vi "Demo - GNU Octave Terminal.vi"() -> ()   [LabVIEW 2020, in "GOLPI library.lvlib"]
doc: "Demontration of GOLPI: GNU Octave terminal.\n\n---\nGOLPI works only with lv_proc.dll library, which is part of vipm package or should be delivered together with packed library. Placement of this dll is selected in terminal of Start GNU Octave.vi."
uses:
  GOLPI library.lvlib
  GOLPI reference Type Def.ctl
  Pipe Handle.ctl
  LV Process library.lvlib
panel:
  in  "hide debug console":bool=TRUE
  out "debug data":T1(array[cluster])
  in  "debug mode\n(only nonempty buffers)":bool
  out "GOLPI ref. pipe":T2={"pipe handle"={"lv_proc.dll file path"=path "", "process instance handle"=[], "debug mode"=FALSE, "debug data"=[]}, "fast read timeout [ms]"=500, "fast read settle time [ms]"=10, "fast read to multiple [ms]"=1, "max elements per input line"=100, "slow read timeout [ms]"=500, "stdin double format specifier"="%_16e", "max elements per stdout output column"=100, "console mode bitstream"=FALSE, "bitstream first read timeout [ms]"=1000, "bitstream read timeout [ms]"=50, "struct transfer possible"=FALSE, "matlab mode"=FALSE}
  out "bytes remaining":i32
  in  "quit":bool
  out "GNU Octave running":bool
  out "read buffer":string
  in  "command buffer":string
  in  "command":bool
  out "objects after start":refnum<vi>[](array[refnum])
  out "objects before start":refnum<vi>[](array[refnum])
  in  "stop":bool
  out "error":errorcluster
  in  "start":bool
  in  "octave binary directory":path=path "C:/Program Files/Octave-3.6.2/bin"
  in  "working directory":path=path "C:/"
  out "exit code":i32
  out "GNU Octave version":string
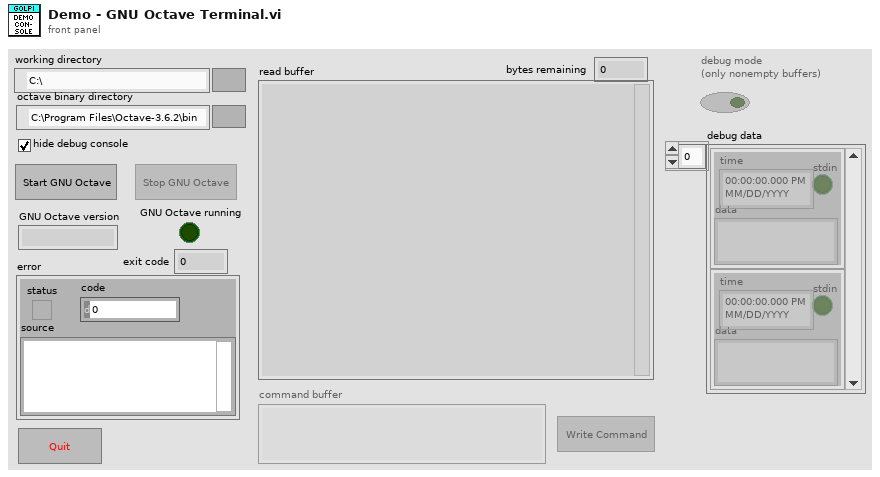
[diagram p1: front panel]
types:
  T1 = cluster{"time":timestamp, "stdin":bool, "data":string}[]
  T2 = typedef "GOLPI library.lvlib/GOLPI reference Type Def.ctl" = cluster{"pipe handle":T3, "fast read timeout [ms]":u32, "fast read settle time [ms]":u32, "fast read to multiple [ms]":u32, "max elements per input line":u32, "slow read timeout [ms]":u32, "stdin double format specifier":string, "max elements per stdout output column":u32, "console mode bitstream":bool, "bitstream first read timeout [ms]":u32, "bitstream read timeout [ms]":u32, "struct transfer possible":bool, "matlab mode":bool}
  T3 = typedef "LV Process library.lvlib/Pipe Handle.ctl" = cluster{"lv_proc.dll file path":path, "process instance handle":u32[], "debug mode":bool, "debug data":cluster{"time":timestamp, "stdin":bool, "data":string}[]}
  T4 = enum8{"Enabled", "Disabled", "Disabled and Grayed Out"}
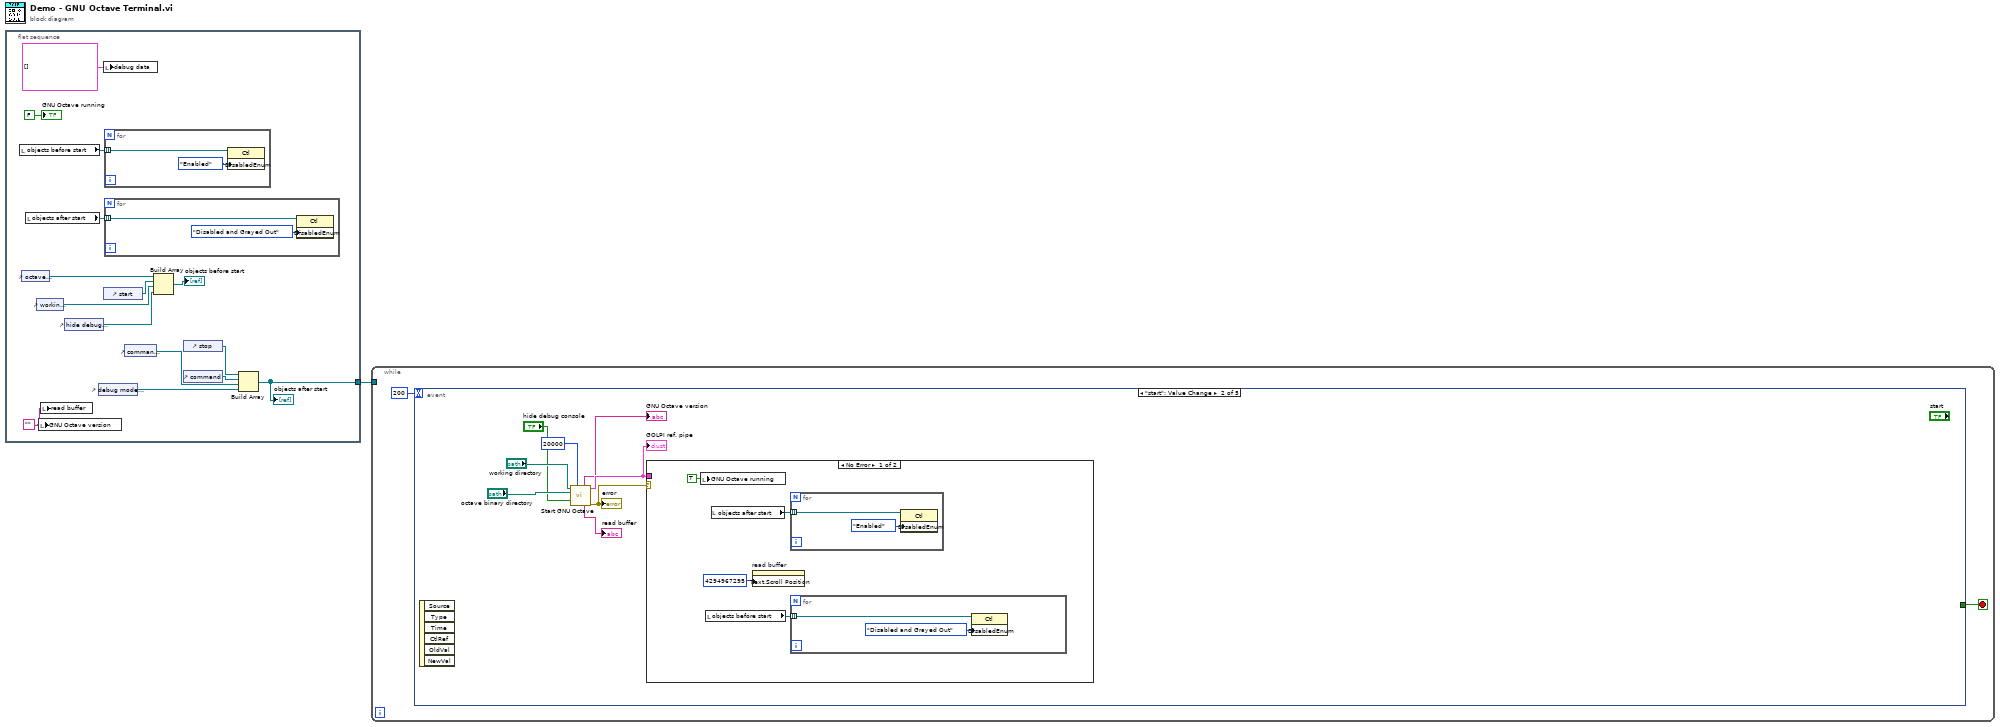
[diagram p0: block diagram]
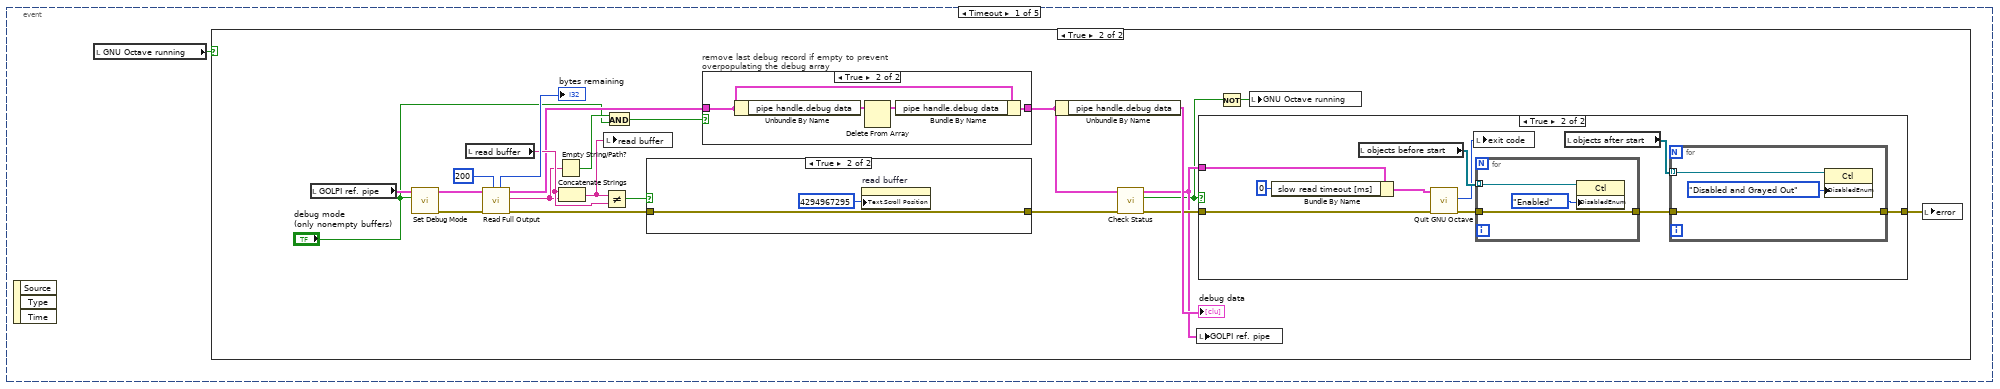
[diagram p2: hidden frame]
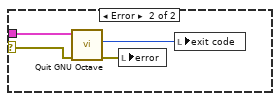
[diagram p7: hidden frame]
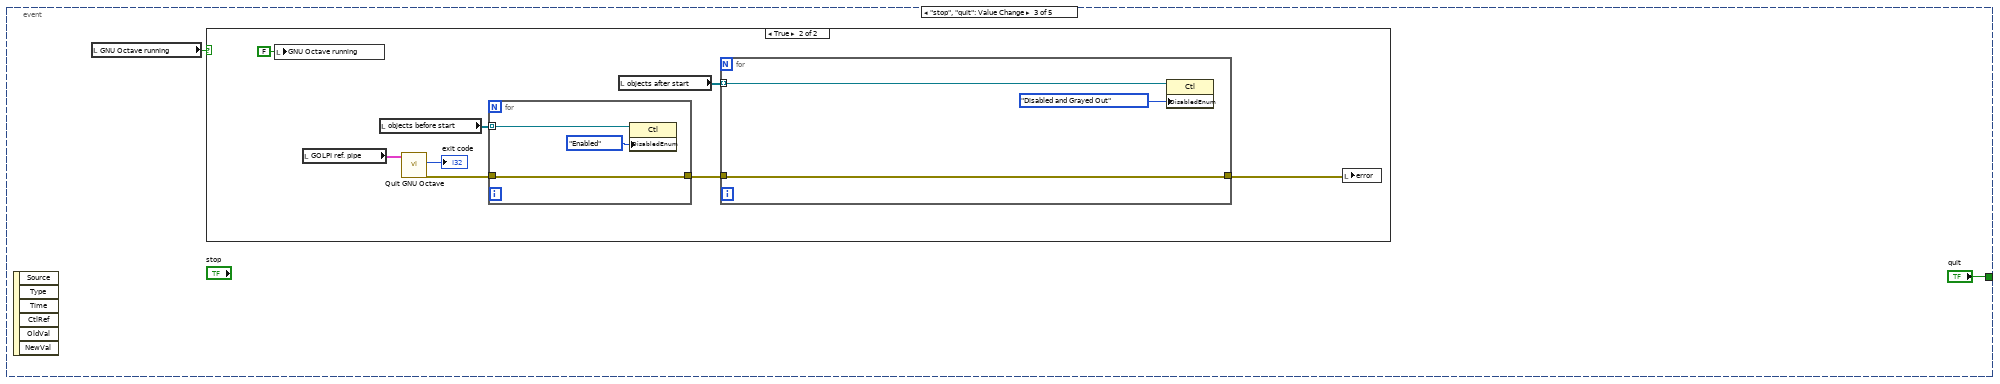
[diagram p8: hidden frame]
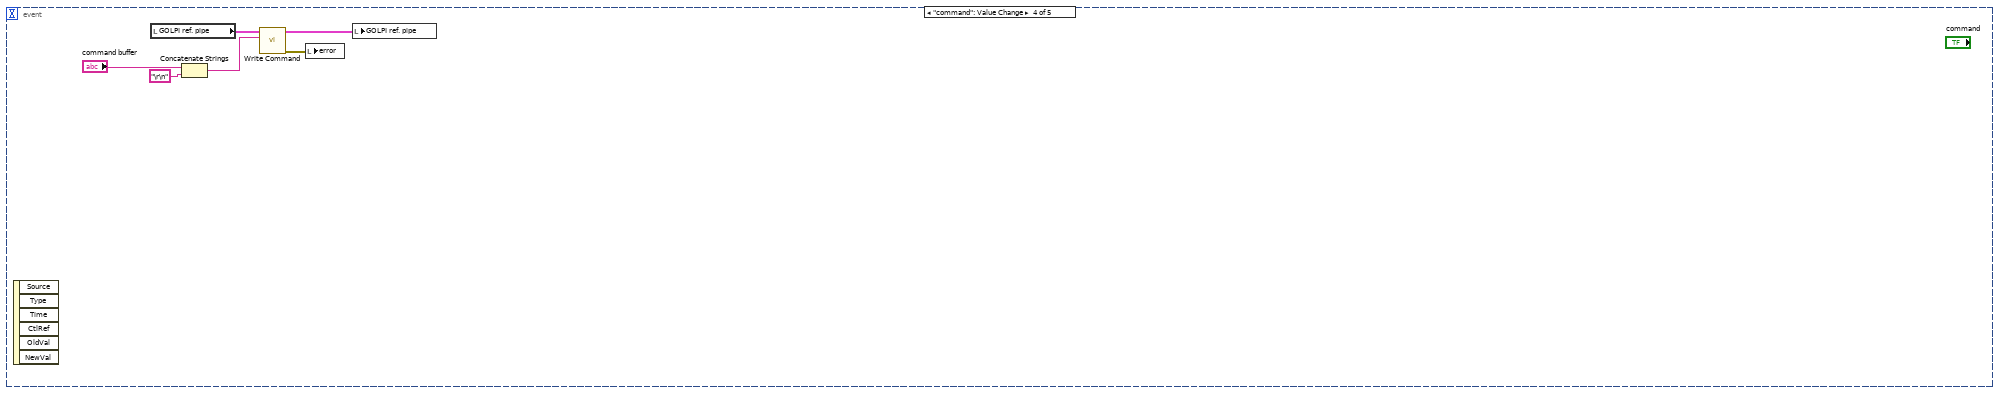
[diagram p10: hidden frame]
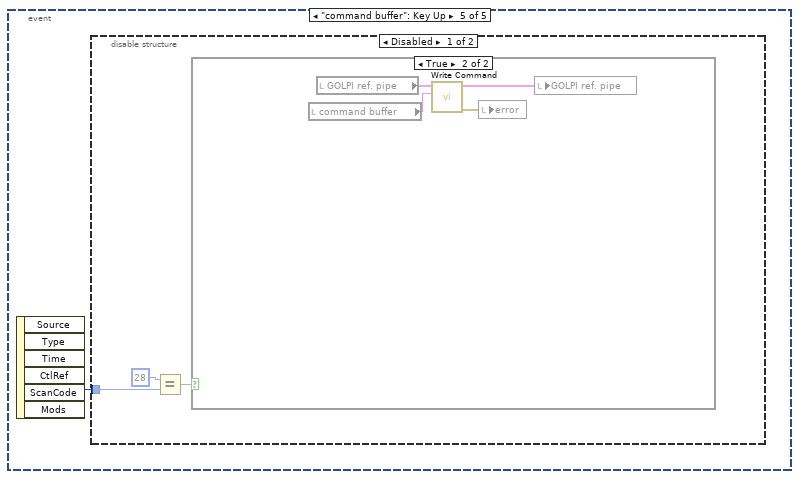
[diagram p11: hidden frame]
diagram:
  n1 = flat-sequence {
    tunnel: [w11] -> w1
    frame #0 {
      w8 = "" ("read buffer")
      n2 = local read "objects before start"() -> (w3:refnum<vi>[])
      n3 = control-ref of="octave binary directory"() -> (w16:refnum<vi>)
      n4 = local read "objects after start"() -> (w4:refnum<vi>[])
      n5 = control-ref of="working directory"() -> (w14:refnum<vi>)
      n6 = local write "GNU Octave version"(w8) -> ()
      n7 = local write "read buffer"(w8) -> ()
      n8 = control-ref of="hide debug console"() -> (w2:refnum<vi>)
      n9 = control-ref of="debug mode\n(only nonempty buffers)"() -> (w6:refnum<vi>)
      n10 = local write "debug data"(T1 [] ("Debug data")) -> ()
      n11 = control-ref of="start"() -> (w15:refnum<vi>)
      n12 = for {
        tunnel: w3 -> [w20] mode=indexing
        n13 = property class="Ctl"(reference=w20, "DisabledEnum"=T4."Enabled" ("Disabled")) -> ()  [unwired: 1 in, 2 out]
      }
      n14 = for {
        tunnel: w4 -> [w18] mode=indexing
        n15 = property class="Ctl"(reference=w18, "DisabledEnum"=T4."Disabled and Grayed Out" ("Disabled")) -> ()  [unwired: 1 in, 2 out]
      }
      n16 = control-ref of="command buffer"() -> (w9:refnum<vi>)
      n17 = Build Array(w16, w15, w14, w2) -> (→"objects before start":refnum<vi>[])
      n18 = control-ref of="stop"() -> (w12:refnum<vi>)
      n19 = control-ref of="command"() -> (w10:refnum<vi>)
      n20 = Build Array(w12, w10, w9, w6) -> (w11:refnum<vi>[])
      "objects after start" <- w11
      "GNU Octave running" <- FALSE ("GNU Octave running")
    }
  }
  n21 = while {
    tunnel: w1 -> [_]
    stop <- w21 stop-if-true
    n22 = event shown="[1] \"start\": Value Change" {
      selector: _ -> [_ _ _ _ _]
      dyn-events: _ -> [_ _ _ _ _]
      timeout: 200 -> [_ _ _ _ _]
      tunnel: [_ _ "quit" _ _] -> w21
      event Timeout {
        n23 = event-data() -> ()  [unwired: 1 in, 3 out]
        n24 = local read "GNU Octave running"() -> (w23:bool)
        n25 = case shown="True" w23 {
          frame False {
          }
          frame True {
            n26 = local read "GOLPI ref. pipe"() -> (w37:T2)
            n27 = call "Set Debug Mode.vi"("debug mode (F)"="debug mode\n(only nonempty buffers)", "GOLPI ref. in"=w37) -> ("error out"=w39:errorcluster, "GOLPI ref. out"=w38:T2)  [unwired: 6 in, 2 out]
            n28 = local read "read buffer"() -> (w41:string)
            n29 = call "Read Full Output.vi"("timeout [ms]"=u32 200, "error in"=w39, "GOLPI ref. in"=w38) -> ("error out"=w45:errorcluster, "read buffer"=w36:string, "GOLPI ref. out"=w35:T2, "bytes remaining"=→"bytes remaining":i32)  [unwired: 5 in]
            n30 = Empty String/Path?(string/path=w36) -> (empty?=w34:bool)
            n31 = Concatenate Strings(w41, w36) -> (w42:string)
            n32 = local write "read buffer"(w42) -> ()
            n33 = Not Equal?(x=w42, y=w41) -> (x != y?=w40:bool)
            n34 = And(x=w34, y="debug mode\n(only nonempty buffers)") -> (x .and. y?=w32:bool)
            n35 = case shown="True" w40 {
              tunnel: [w68 w69] -> w29
              tunnel: w45 -> [w68 w69]
              frame False {
              }
              frame True {
                n36 = property on="read buffer" class="Str"("Text.Scroll Position"=u32 4294967295) -> ()  [unwired: 2 in, 2 out]
              }
            }
            n37 = case "remove last debug record if empty to prevent overpopulating the debug array" shown="True" w32 {
              tunnel: w35 -> [w63 w67]
              tunnel: [w63 w66] -> w30
              frame False {
              }
              frame True {
                n38 = Unbundle By Name(w67) -> ("pipe handle.debug data"=w64:T1)
                n39 = Delete From Array(array=w64) -> (array with subset deleted=w65:T1)  [unwired: 2 in, 1 out]
                n40 = Bundle By Name(cluster=w67, "pipe handle.debug data"=w65) -> (w66:T2)
              }
            }
            n41 = Unbundle By Name(w30) -> ("pipe handle.debug data"=→"debug data":T1)
            n42 = call "Check Status.vi"("error in"=w29, "GOLPI ref. in"=w30) -> ("error out"=w28:errorcluster, "exited?"=w25:bool, "GOLPI ref. out"=w26:T2)  [unwired: 7 in]
            n43 = local write "GOLPI ref. pipe"(w26) -> ()
            n44 = case shown="True" w25 {
              tunnel: w28 -> [w46 w54]
              tunnel: [w46 w53] -> w27
              tunnel: w26 -> [_ w49]
              frame False {
              }
              frame True {
                n45 = Bundle By Name(cluster=w49, "slow read timeout [ms]"=u32 0) -> (w47:T2)
                n46 = local read "objects before start"() -> (w52:refnum<vi>[])
                n47 = call "Quit GNU Octave.vi"("error in"=w54, "GOLPI ref. in"=w47) -> ("error out"=w56:errorcluster, "exit code"=w50:i32)  [unwired: 8 in]
                n48 = local write "exit code"(w50) -> ()
                n49 = for {
                  tunnel: w52 -> [w62] mode=indexing
                  tunnel: w56 -> [w60]
                  tunnel: [w60] -> w55
                  n50 = property class="Ctl"(reference=w62, "DisabledEnum"=T4."Enabled" ("Disabled")) -> ()  [unwired: 1 in, 2 out]
                }
                n51 = local read "objects after start"() -> (w51:refnum<vi>[])
                n52 = for {
                  tunnel: w51 -> [w59] mode=indexing
                  tunnel: [w57] -> w53
                  tunnel: w55 -> [w57]
                  n53 = property class="Ctl"(reference=w59, "DisabledEnum"=T4."Disabled and Grayed Out" ("Disabled")) -> ()  [unwired: 1 in, 2 out]
                }
              }
            }
            n54 = Not(x=w25) -> (.not. x?=w24:bool)
            n55 = local write "GNU Octave running"(w24) -> ()
            n56 = local write "error"(w27) -> ()
          }
        }
      }
      event "start": Value Change {
        n57 = event-data() -> ()  [unwired: 1 in, 6 out]
        n58 = call "Start GNU Octave.vi"("working dir (user home)"="working directory", "full start timeout [ms] (20000)"=u32 20000 ("full start timeout [ms] (5000)"), "octave binary file or dir (autofind)"="octave binary directory", "hide debug console (T)"="hide debug console") -> ("GNU Octave version"=→"GNU Octave version":string, "GOLPI ref. out"=w75:T2, "initial output"=→"read buffer":string, "error out"=w76:errorcluster)  [unwired: 8 in]
        "error" <- w76
        "GOLPI ref. pipe" <- w75
        n59 = case shown="No Error" w76 {
          selector: w76 -> [_ w88]
          tunnel: w75 -> [_ w90]
          frame No Error {
            n60 = local write "GNU Octave running"(TRUE ("GNU Octave running")) -> ()
            n61 = local read "objects before start"() -> (w82:refnum<vi>[])
            n62 = local read "objects after start"() -> (w81:refnum<vi>[])
            n63 = property on="read buffer" class="Str"("Text.Scroll Position"=u32 4294967295) -> ()  [unwired: 2 in, 2 out]
            n64 = for {
              tunnel: w81 -> [w84] mode=indexing
              n65 = property class="Ctl"(reference=w84, "DisabledEnum"=T4."Enabled" ("Disabled")) -> ()  [unwired: 1 in, 2 out]
            }
            n66 = for {
              tunnel: w82 -> [w86] mode=indexing
              n67 = property class="Ctl"(reference=w86, "DisabledEnum"=T4."Disabled and Grayed Out" ("Disabled")) -> ()  [unwired: 1 in, 2 out]
            }
          }
          frame Error {
            n68 = call "Quit GNU Octave.vi"("error in"=w88, "GOLPI ref. in"=w90) -> ("error out"=w87:errorcluster, "exit code"=w89:i32)  [unwired: 8 in]
            n69 = local write "error"(w87) -> ()
            n70 = local write "exit code"(w89) -> ()
          }
        }
      }
      event "stop", "quit": Value Change {
        n71 = event-data() -> ()  [unwired: 1 in, 6 out]
        n72 = local read "GNU Octave running"() -> (w91:bool)
        n73 = case shown="True" w91 {
          frame False {
          }
          frame True {
            n74 = local write "GNU Octave running"(FALSE ("GNU Octave running")) -> ()
            n75 = local read "GOLPI ref. pipe"() -> (w96:T2)
            n76 = local read "objects before start"() -> (w99:refnum<vi>[])
            n77 = call "Quit GNU Octave.vi"("GOLPI ref. in"=w96) -> ("error out"=w95:errorcluster, "exit code"=→"exit code":i32)  [unwired: 9 in]
            n78 = for {
              tunnel: w99 -> [w106] mode=indexing
              tunnel: w95 -> [w104]
              tunnel: [w104] -> w94
              n79 = property class="Ctl"(reference=w106, "DisabledEnum"=T4."Enabled" ("Disabled")) -> ()  [unwired: 1 in, 2 out]
            }
            n80 = local read "objects after start"() -> (w98:refnum<vi>[])
            n81 = for {
              tunnel: w98 -> [w103] mode=indexing
              tunnel: [w101] -> w93
              tunnel: w94 -> [w101]
              n82 = property class="Ctl"(reference=w103, "DisabledEnum"=T4."Disabled and Grayed Out" ("Disabled")) -> ()  [unwired: 1 in, 2 out]
            }
            n83 = local write "error"(w93) -> ()
          }
        }
      }
      event "command": Value Change {
        n84 = event-data() -> ()  [unwired: 1 in, 6 out]
        n85 = local read "GOLPI ref. pipe"() -> (w112:T2)
        n86 = Concatenate Strings("command buffer", "\r\n") -> (w107:string)
        n87 = call "Write Command.vi"("command"=w107, "GOLPI ref. in"=w112) -> ("error out"=w111:errorcluster, "GOLPI ref. out"=w110:T2)  [unwired: 8 in]
        n88 = local write "error"(w111) -> ()
        n89 = local write "GOLPI ref. pipe"(w110) -> ()
      }
      event "command buffer": Key Up {
        n90 = event-data() -> ("ScanCode"=w113:i16)  [unwired: 1 in, 5 out]
        n91 = disable-structure shown="Disabled" {
          disable-tunnel: w113 -> [w115 _]
          frame Disabled {
            n92 = Equal?(x=i16 28, y=w115) -> (x = y?=w116:bool)
            n93 = case shown="True" w116 {
              frame False {
              }
              frame True {
                n94 = local read "command buffer"() -> (w120:string)
                n95 = local read "GOLPI ref. pipe"() -> (w117:T2)
                n96 = call "Write Command.vi"("command"=w120, "GOLPI ref. in"=w117) -> ("error out"=w118:errorcluster, "GOLPI ref. out"=w119:T2)  [unwired: 8 in]
                n97 = local write "error"(w118) -> ()
                n98 = local write "GOLPI ref. pipe"(w119) -> ()
              }
            }
          }
          frame Enabled {
          }
        }
      }
    }
  }
